vi "Test Flatten.vi"() -> ()   [LabVIEW 2021]
uses:
  CIF_NIChn_Fifo_Power_DVR.lvclass
  ChannelCommon/typedef/FIFO Header.ctl
  ChannelCommon/ChannelCommon.lvlib
  ChannelCommon/typedef/Datatype Waveform.ctl
  ChannelCommon/typedef/TimeStamps.ctl
panel:
  in  "FIFO Timestamps":T1
  out "Data out":T2[](array[typedef])
  in  "Data In":T2[](array[typedef])=[{"measurement"=[0.0, 0.0, 0.0, 0.0, 0.0, 0.0, 0.0, 3.14], "dT"=0.01, "Timestamp"=498, "Read Lock"=FALSE}, {"measurement"=[0.0, 0.0, 0.0, 0.0, 0.0, 0.0, 0.0, 9.8], "dT"=0.12, "Timestamp"=12345, "Read Lock"=FALSE}]
  out "Header":T3={"Length"=52, "T0"=321, "T_Out"=123, "T_Tx"=1724093393726059437, "Ctr"=1, "ClockID"=0}
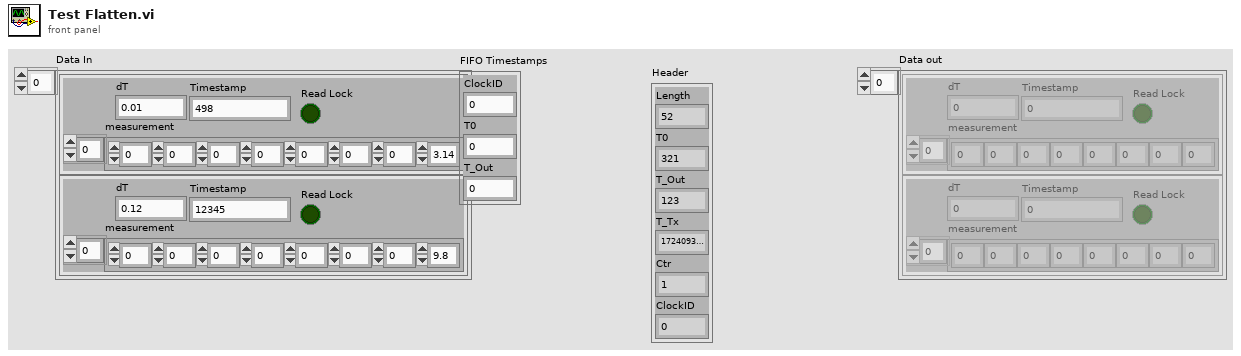
[diagram p1: front panel]
types:
  T1 = typedef "ChannelCommon.lvlib/TimeStamps.ctl" = cluster{"ClockID":u8, "T0":u64, "T_Out":u64}
  T2 = typedef "ChannelCommon.lvlib/Datatype Waveform.ctl" = cluster{"measurement":dbl[], "dT":dbl, "Timestamp":u64, "Read Lock":bool}
  T3 = typedef "ChannelCommon.lvlib/FIFO Header.ctl" = cluster{"Length":u64, "T0":i64, "T_Out":i64, "T_Tx":i64, "Ctr":u64, "ClockID":u8}
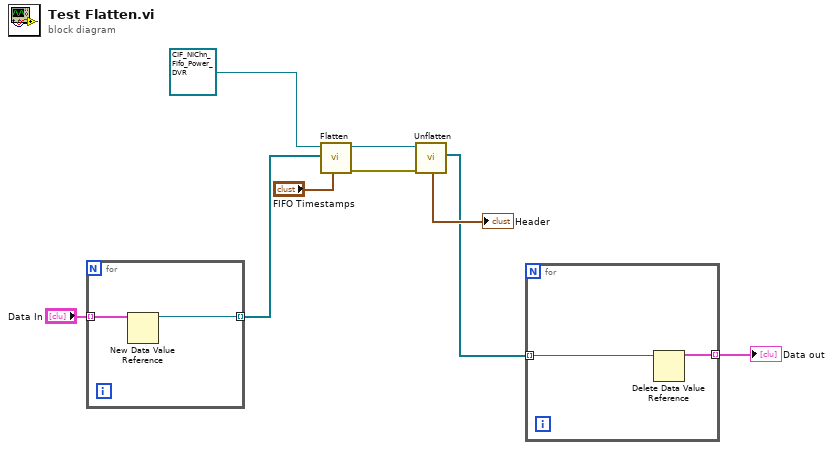
[diagram p0: block diagram]
diagram:
  n1 = for {
    tunnel: "Data In" -> [w11] mode=indexing
    tunnel: [w10] -> w3 mode=indexing
    n2 = New Data Value Reference(data value=w11) -> (data value reference=w10:refnum<data-value>)  [unwired: 1 in, 1 out]
  }
  n3 = call "Flatten.vi"("FIFO Timestamps"="FIFO Timestamps", "Data In"=w3, "CIFTag in"=refnum<class "CIF_NIChn_Fifo_Power_DVR.lvclass"> refnum ("CIF_NIChn_Fifo_Power.lvclass")) -> ("error out"=w8:errorcluster, "CIFTag out"=w9:refnum<class "CIF_NIChn_Fifo_Power_DVR.lvclass">)  [unwired: 6 in, 1 out]
  n4 = call "Unflatten.vi"("error in (no error)"=w8, "CIFFifoCAN in"=w9) -> ("Data Out"=w2:refnum<data-value>[], "Header"=→"Header":T3)  [unwired: 6 in, 2 out]
  n5 = for {
    tunnel: w2 -> [w12] mode=indexing
    tunnel: [w13] -> w1 mode=indexing
    n6 = Delete Data Value Reference(data value reference=w12) -> (data value=w13:T2)  [unwired: 1 in, 1 out]
  }
  "Data out" <- w1
